vi "Configure Source.vi"(8 "error in (no error)":errorcluster, 10 "Source (F:Volt)":bool, 11 "Power Supply in":refnum<class "Power Supply.lvclass">) -> (0 "error out":errorcluster, 3 "Power Supply out":refnum<class "Power Supply.lvclass">)   [LabVIEW 2020, in "Power Supply.lvclass"]
uses:
  Power Supply.lvclass
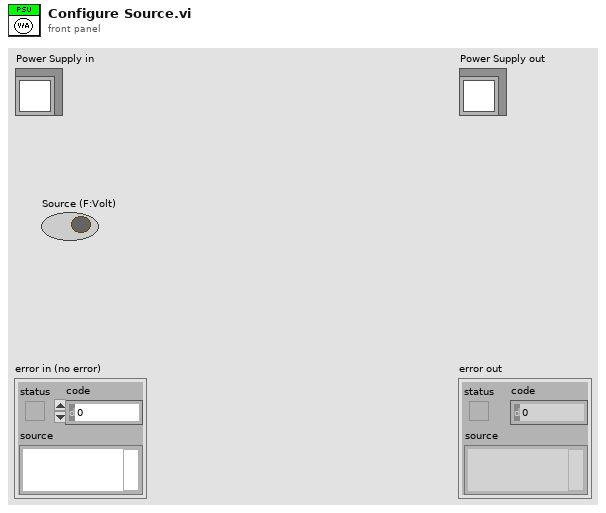
[diagram p1: front panel]
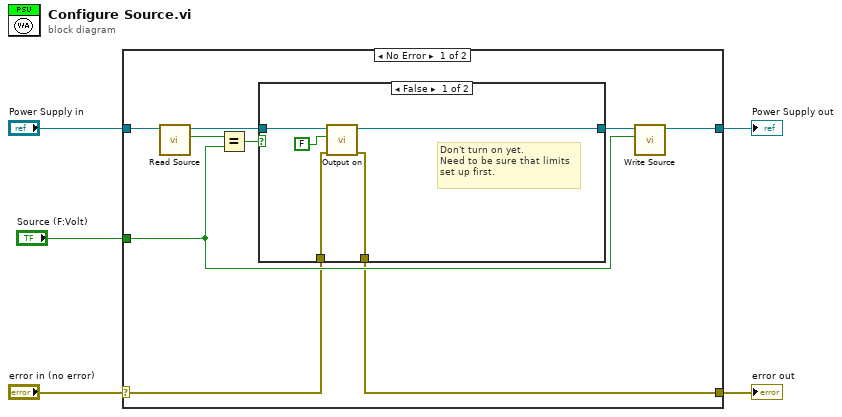
[diagram p0: block diagram]
diagram:
  n1 = case shown="No Error" "error in (no error)" {
    selector: "error in (no error)" -> [w7 w23]
    tunnel: [w6 w23] -> w2
    tunnel: [w14 w22] -> w1
    tunnel: "Power Supply in" -> [w8 w22]
    tunnel: "Source (F:Volt)" -> [w12 _]
    frame No Error {
      n2 = call-dynamic "Read Source.vi"("Power Supply in"=w8) -> ("Source"=w13:bool, "Power Supply out"=w10:refnum<class "Power Supply.lvclass">)  [unwired: 9 in]
      n3 = Equal?(x=w13, y=w12) -> (x = y?=w11:bool)
      n4 = case shown="False" w11 {
        tunnel: w10 -> [w19 w21]
        tunnel: [w17 w21] -> w9
        tunnel: w7 -> [w16 w20]
        tunnel: [w15 w20] -> w6
        frame False {
          # "Don't turn on yet.\nNeed to be sure that limits\nset up first."
          n5 = call-dynamic "Output on.vi"("error in (no error)"=w16, "Output On"=FALSE, "Power Supply in"=w19) -> ("error out"=w15:errorcluster, "Power Supply out"=w17:refnum<class "Power Supply.lvclass">)  [unwired: 7 in]
        }
        frame True {
          # "No change"
        }
      }
      n6 = call-dynamic "Write Source.vi"("Source"=w12, "Power Supply in"=w9) -> ("Power Supply out"=w14:refnum<class "Power Supply.lvclass">)  [unwired: 9 in]
    }
    frame Error {
    }
  }
  "error out" <- w2
  "Power Supply out" <- w1
